vi "Format Target Information for Dialog.vi"(11 "target settings in":T1={"Hostname"="", "Serial number"="", "Product name"="", "Product code"=0, "System status"="", "Credential type"=enum."None/Unlocked", "User added?"=FALSE, "Primary NIC"={"MAC address"="", "IP Address Request Mode"=2, "IP address"="", "Subnet mask"="", "Gateway"="", "DNS server"=""}, "System Credentials"={"Username"="", "Password"=""}} {"Primary NIC"."IP Address Request Mode" items=["Static"=1, "DHCP/Link-Local"=2, "Link-Local Only"=4, "DHCP Only"=8]}) -> (0 "Target Information":string[][](array[string]), 3 "target settings out":T1={"Hostname"="", "Serial number"="", "Product name"="", "Product code"=0, "System status"="", "Credential type"=enum."None/Unlocked", "User added?"=FALSE, "Primary NIC"={"MAC address"="", "IP Address Request Mode"=2, "IP address"="", "Subnet mask"="", "Gateway"="", "DNS server"=""}, "System Credentials"={"Username"="", "Password"=""}} {"Primary NIC"."IP Address Request Mode" items=["Static"=1, "DHCP/Link-Local"=2, "Link-Local Only"=4, "DHCP Only"=8]})   [LabVIEW 2020]
uses:
  Controls/Target Information.ctl
  Controls/Target Network Settings.ctl
  Controls/System Credentials.ctl
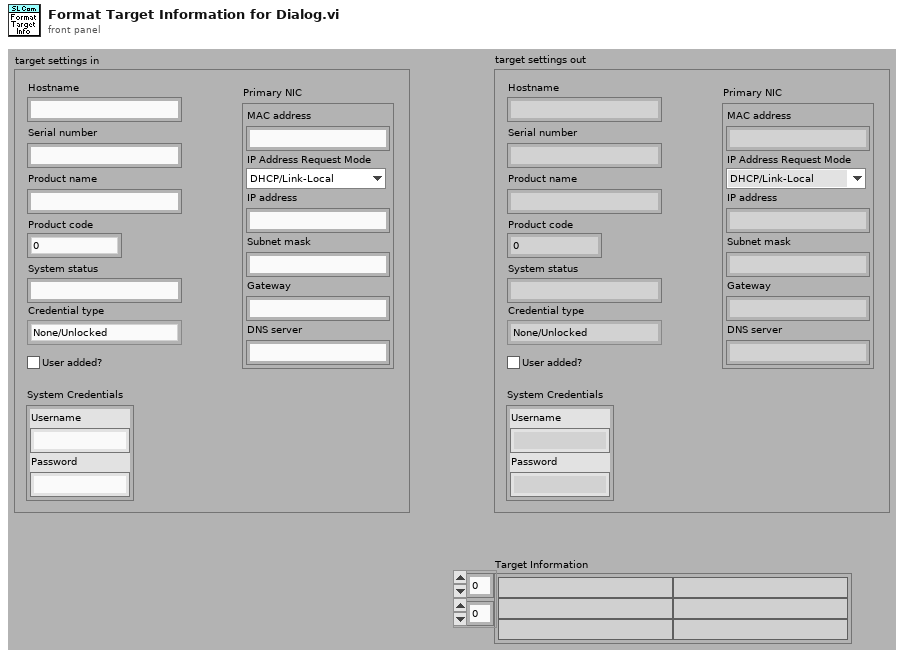
[diagram p1: front panel]
types:
  T1 = typedef "Target Information.ctl" = cluster{"Hostname":string, "Serial number":string, "Product name":string, "Product code":i32, "System status":string, "Credential type":enum16{"None/Unlocked", "FTP Password", "NIAuth Credentials"}, "User added?":bool, "Primary NIC":T2, "System Credentials":T3}
  T2 = typedef "Target Network Settings.ctl" = cluster{"MAC address":string, "IP Address Request Mode":i32, "IP address":string, "Subnet mask":string, "Gateway":string, "DNS server":string}
  T3 = typedef "System Credentials.ctl" = cluster{"Username":string, "Password":string}
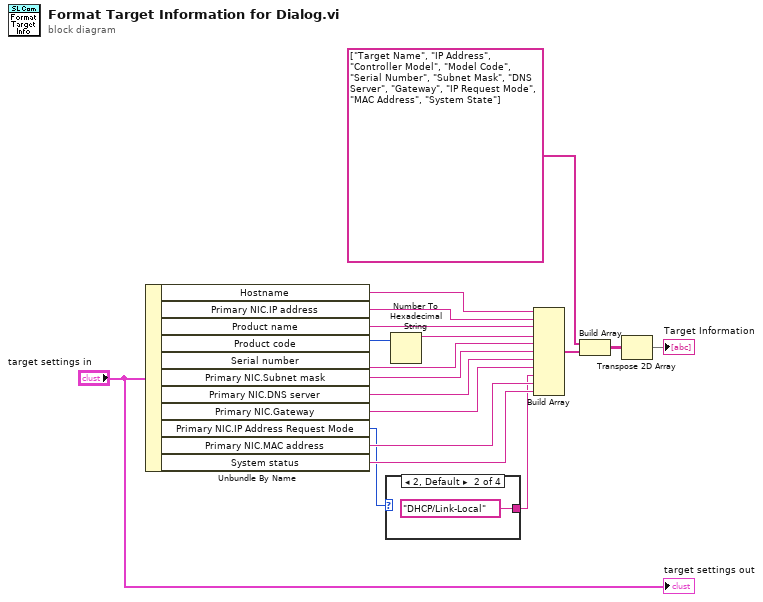
[diagram p0: block diagram]
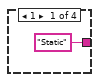
[diagram p2: hidden frame]
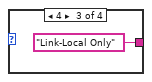
[diagram p3: hidden frame]
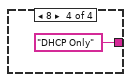
[diagram p4: hidden frame]
diagram:
  n1 = Unbundle By Name("target settings in") -> ("Hostname"=w14:string, "Primary NIC.IP address"=w13:string, "Product name"=w12:string, "Product code"=w11:i32, "Serial number"=w9:string, "Primary NIC.Subnet mask"=w8:string, "Primary NIC.DNS server"=w7:string, "Primary NIC.Gateway"=w6:string, "Primary NIC.IP Address Request Mode"=w3:i32, "Primary NIC.MAC address"=w5:string, "System status"=w4:string)
  n2 = case shown="2, Default" w3 {
    tunnel: ["Static" "DHCP/Link-Local" "Link-Local Only" "DHCP Only"] -> w2
    frame 1 {
    }
    frame 2, Default {
    }
    frame 4 {
    }
    frame 8 {
    }
  }
  n3 = Number To Hexadecimal String(2:w11) -> (0:w10:string)  [unwired: 1 in]
  n4 = Build Array(w14, w13, w12, w10, w9, w8, w7, w6, w2, w5, w4) -> (w18:string[])
  n5 = Build Array(string[] ["Target Name", "IP Address", "Controller Model", "Model Code", "Serial Number", "Subnet Mask", "DNS Server", "Gateway", "IP Request Mode", "MAC Address", "System State"] ("element"), w18) -> (w16:string[][])
  n6 = Transpose 2D Array(2D array=w16) -> (transposed array=→"Target Information":string[][])
  "target settings out" <- "target settings in"
